vi "Sonar_test.vi"() -> ()   [LabVIEW 2018]
uses:
  <userlib>/_OpenG.lib/comparison/comparison.llb/Boolean Changed__ogtk.vi
panel:
  in  "Distance":i32
  out "Angle":i32
  in  "Sweep":bool
  out "Polar Plot":picture
  in  "Stop button":bool
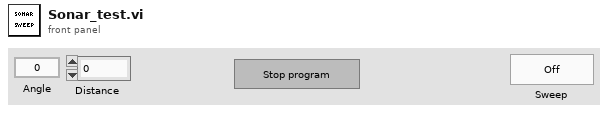
[diagram p1: front panel]
types:
  T1 = cluster{"maximum":dbl, "minimum":dbl, "clip to min":bool, "log?(F)":bool, "grid color":u32, "plot color":u32, "fmt and prec":cluster{"format":enum8{"Decimal", "Scientific", "Engineering", "Binary", "Octal", "Hex"}, "precision":u8}, "visible section":u16}
  T2 = typedef "imagedata.ctl" = cluster{"image type":i32, "image depth":i32, "image":u8[], "mask":u8[], "colors":u32[], "Rectangle":cluster{"left":i16, "top":i16, "right":i16, "bottom":i16}}
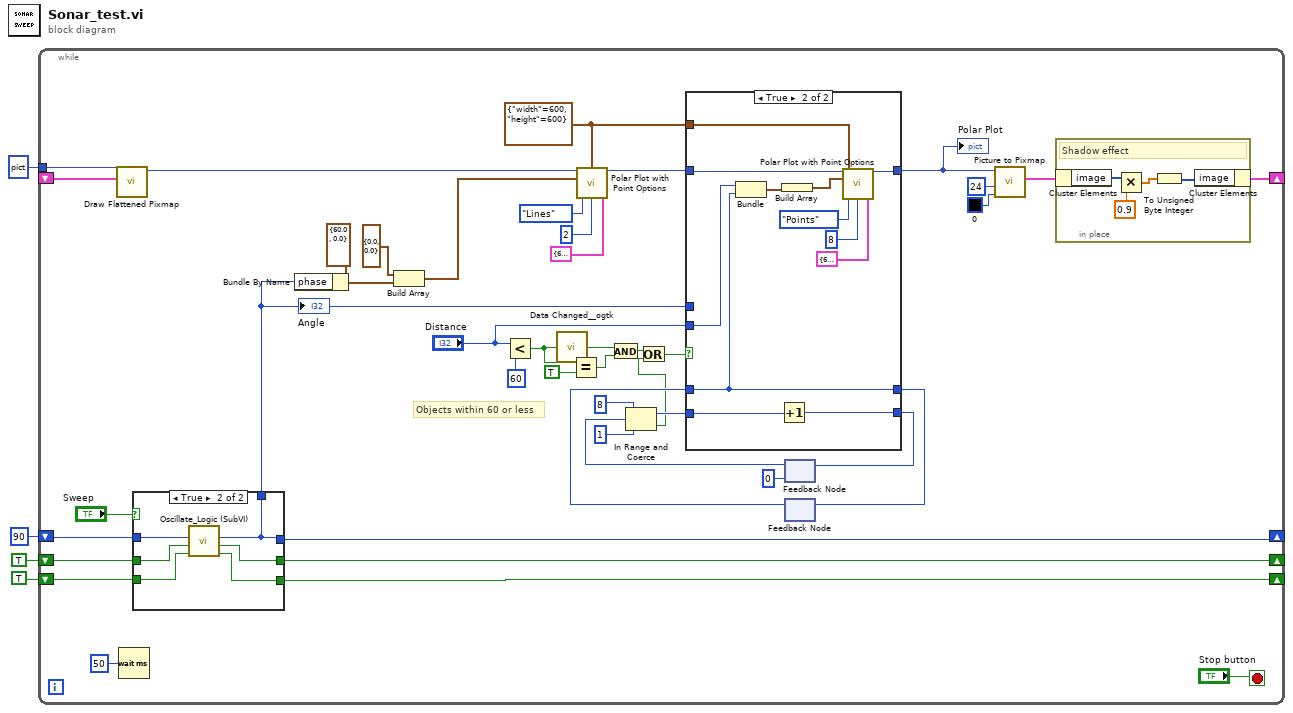
[diagram p0: block diagram]
diagram:
  n1 = while {
    shift-right: [w40] -> _
    shift-left: 90 -> [w41]
    shift-right: [w42] -> _
    shift-left: TRUE -> [w45]
    shift-right: [w43] -> _
    shift-left: TRUE -> [w44]
    shift-right: [w36] -> _
    shift-left: _ -> [w33]
    tunnel: picture data[5B] ("2D Picture") -> [w31]
    stop <- "Stop button" stop-if-true
    w21 = cluster{"width":i16, "height":i16} {"width"=600, "height"=600} ("dimensions (w,h)")
    # "Objects within 60 or less"
    n2 = call <vilib>:"Draw Flattened Pixmap.vi"("image data"=w33, "picture"=w31) -> ("new picture"=w32:picture)  [unwired: 7 in]
    n3 = Wait (ms)(milliseconds to wait=u32 50 ("Speed")) -> ()  [unwired: 1 out]
    n4 = case shown="True" "Sweep" {
      tunnel: w45 -> [w69 w70]
      tunnel: w44 -> [w68 w71]
      tunnel: [w68 w73] -> w43
      tunnel: [w69 w72] -> w42
      tunnel: w41 -> [w67 w75]
      tunnel: [w67 w74] -> w40
      tunnel: [w67 w74] -> w24
      frame False {
      }
      frame True {
        n5 = call "Oscillate_Logic (SubVI).vi"("Boolearn Input 2"=w71, "Boolean Input 1"=w70, "Numeric in"=w75) -> ("Boolean Output 2"=w73:bool, "Boolean Output 1"=w72:bool, "Numeric out"=w74:i32)  [unwired: 6 in]
      }
    }
    "Angle" <- w24
    n6 = Bundle By Name(cluster=cluster{"magnitude":dbl, "phase":dbl} {"magnitude"=60.0, "phase"=0.0} ("Cluster 2"), "phase"=w24) -> (w28:cluster{"magnitude":dbl, "phase":dbl})
    n7 = Build Array(cluster{"magnitude":dbl, "phase":dbl} {"magnitude"=0.0, "phase"=0.0} ("Cluster 2"), w28) -> (w26:cluster{"magnitude":dbl, "phase":dbl}[])
    n8 = Less?(x="Distance", y=60) -> (x < y?=w7:bool)
    n9 = call-poly <userlib>:"Data Changed__ogtk.vi"("Boolean"=w7) -> ("Changed"=w12:bool)
    n10 = Equal?(x=w7, y=TRUE) -> (x = y?=w13:bool)
    n11 = call <vilib>:"Polar Plot with Point Options.vi"("picture"=w32, "data array [mag, phase (deg)]"=w26, "dimensions (w,h)"=w21, "polar attributes"=T1 {"maximum"=60.0, "minimum"=0.0, "clip to min"=FALSE, "log?(F)"=FALSE, "grid color"=6710886, "plot color"=65280, "fmt and prec"={"format"=enum."Decimal", "precision"=0}, "visible section"=8}, "Lines/Points"=enum16{"Lines", "Points"}."Lines", "Size"=u16 2) -> ("new picture"=w25:picture)  [unwired: 9 in]
    n12 = And(x=w12, y=w13) -> (x .and. y?=w10:bool)
    n13 = feedback #1(u8 0) -> (w14:u8)
    n14 = In Range and Coerce(upper limit=u8 8 ("y"), x=w14, lower limit=u8 1) -> (coerced(x)=w15:u8, In Range?=w8:bool)
    n15 = Or(x=w10, y=w8) -> (x .or. y?=w9:bool)
    n16 = feedback #2() -> (w22:i32)  [unwired: 1 in]
    n17 = case shown="True" w9 {
      tunnel: w25 -> [w49 w55]
      tunnel: w24 -> [w50 _]
      tunnel: [w50 w51] -> w23
      tunnel: w22 -> [_ w51]
      tunnel: w21 -> [_ w52]
      tunnel: [w49 w56] -> w20
      tunnel: [_ w61] -> w18
      tunnel: w15 -> [_ w62]
      tunnel: "Distance" -> [_ w53]
      frame False {
      }
      frame True {
        n18 = Bundle("Distance"=w53, "Numeric out"=w51) -> (w60:cluster{"Distance":i32, "Numeric out":i32})  [unwired: 1 in]
        n19 = Increment(x=w62) -> (x+1=w61:u8)
        n20 = Build Array(w60) -> (w54:cluster{"Distance":i32, "Numeric out":i32}[])
        n21 = call <vilib>:"Polar Plot with Point Options.vi"("picture"=w55, "data array [mag, phase (deg)]"=w54, "dimensions (w,h)"=w52, "polar attributes"=T1 {"maximum"=60.0, "minimum"=0.0, "clip to min"=FALSE, "log?(F)"=FALSE, "grid color"=6710886, "plot color"=16711680, "fmt and prec"={"format"=enum."Decimal", "precision"=0}, "visible section"=8}, "Lines/Points"=enum16{"Lines", "Points"}."Points", "Size"=u16 8) -> ("new picture"=w56:picture)  [unwired: 9 in]
      }
    }
    "Polar Plot" <- w20
    n22 = feedback-in #1(w18) -> ()
    n23 = feedback-in #2(w23) -> ()
    n24 = call <vilib>:"Picture to Pixmap.vi"("Background Color"=u32 0, "depth"=24, "picture"=w20) -> ("image data"=w37:T2)  [unwired: 7 in, 1 out]
    n25 = in-place {
      # "Shadow effect"
      n26 = in-place-cluster #3(w37) -> ("image"=w66:u8[])
      n27 = Multiply(x=w66, y=0.9) -> (x*y=w64:dbl[])
      n28 = To Unsigned Byte Integer(number=w64) -> (unsigned 8bit integer=w63:u8[])
      n29 = in-place-cluster #3("image"=w63) -> (w36:T2)
    }
  }
